vi "stations copy Station.vi"(7 "Connection Refnum":T1, 8 "error in (no error)":errorcluster, 9 "Stations Instruments":cluster{"Station Instruments":T2[]}[](array[cluster]), 10 "All Stations (empty)":T3[](array[typedef]), 11 "Station ID to Copy (\"\")":string) -> (0 "error out":errorcluster, 1 "Station Instruments":T2[](array[typedef]), 2 "Station Record":T3, 5 "Connection Refnum":T1)   [LabVIEW 2011]
uses:
  server/database/Stations/Station Record.ctl
  server/database/Stations/Instruments/Instrument Record.ctl
  Summitek EXT/ODBC/SQL Controls/Connection Refnum.ctl
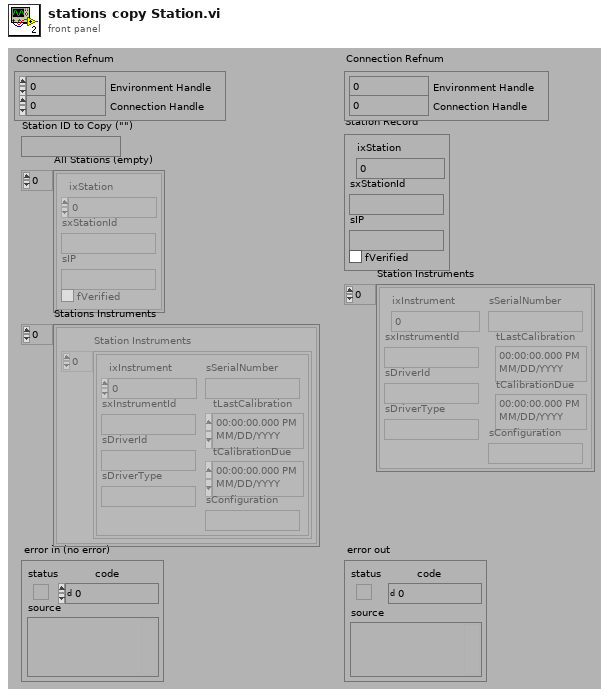
[diagram p1: front panel]
types:
  T1 = typedef "Connection Refnum.ctl" = cluster{"Environment Handle":i32, "Connection Handle":i32}
  T2 = typedef "Instrument Record.ctl" = cluster{"ixInstrument":i32, "sxInstrumentId":string, "sDriverId":string, "sDriverType":string, "sSerialNumber":string, "tLastCalibration":timestamp, "tCalibrationDue":timestamp, "sConfiguration":string}
  T3 = typedef "Station Record.ctl" = cluster{"ixStation":i32, "sxStationId":string, "sIP":string, "fVerified":bool}
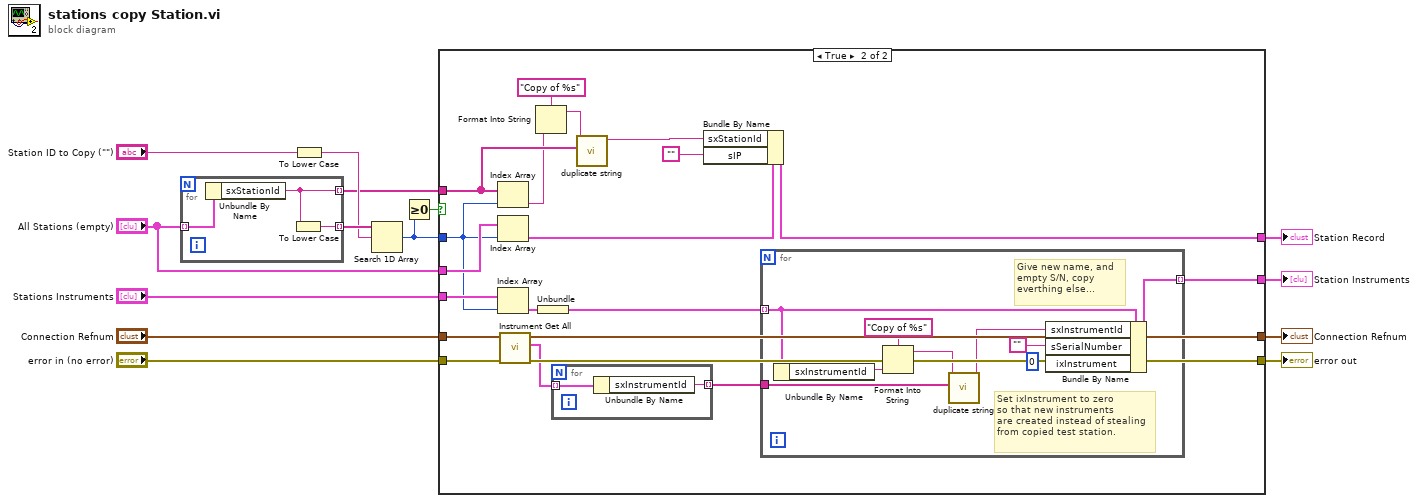
[diagram p0: block diagram]
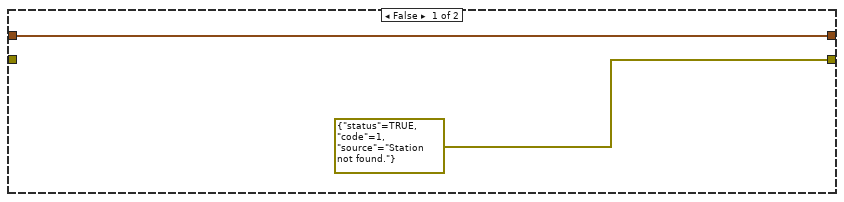
[diagram p2: hidden frame]
diagram:
  n1 = for {
    tunnel: "All Stations (empty)" -> [w17] mode=indexing
    tunnel: [w16] -> w14 mode=indexing
    tunnel: [w15] -> w4 mode=indexing
    n2 = Unbundle By Name(w17) -> ("sxStationId"=w15:string)
    n3 = To Lower Case(string=w15) -> (all lower case string=w16:string)
  }
  n4 = To Lower Case(string="Station ID to Copy (\"\")") -> (all lower case string=w13:string)
  n5 = Search 1D Array(1D array=w14, element=w13) -> (index of element=w11:i32)  [unwired: 1 out]
  n6 = Greater Or Equal To 0?(x=w11) -> (x >= 0?=w10:bool)
  n7 = case shown="True" w10 {
    tunnel: "All Stations (empty)" -> [_ w39]
    tunnel: w11 -> [_ w29]
    tunnel: [_ w37] -> w9
    tunnel: "error in (no error)" -> [_ w27]
    tunnel: [errorcluster {"status"=TRUE, "code"=1, "source"="Station not found."} ("error in (no error)") w26] -> w7
    tunnel: w4 -> [_ w34]
    tunnel: "Stations Instruments" -> [_ w30]
    tunnel: "Connection Refnum" -> [w18 w25]
    tunnel: [w18 w24] -> w2
    tunnel: [_ w20] -> w1
    frame False {
    }
    frame True {
      n8 = Index Array(array=w34, index=w29) -> (element=w33:string)
      n9 = Index Array(array=w39, index=w29) -> (element=w38:T3)
      n10 = Index Array(array=w30, index=w29) -> (element=w28:cluster{"Station Instruments":T2[]})
      n11 = call "Instrument Get All.vi"("error in (no error)"=w27, "Connection Refnum"=w25) -> ("error out"=w26:errorcluster, "Instruments"=w22:T2[], "Connection Refnum"=w24:T1)  [unwired: 2 in, 5 out]
      n12 = Format Into String(format string="Copy of %s", w33) -> (resulting string=w36:string)  [unwired: 2 in, 1 out]
      n13 = Unbundle(w28) -> ("Station Instruments"=w23:T2[])
      n14 = for {
        tunnel: w22 -> [w41] mode=indexing
        tunnel: [w40] -> w21 mode=indexing
        n15 = Unbundle By Name(w41) -> ("sxInstrumentId"=w40:string)
      }
      n16 = call "duplicate string.vi"("Array of Strings"=w34, "String"=w36) -> ("Updated String"=w32:string)  [unwired: 9 out]
      n17 = Bundle By Name(cluster=w38, "sxStationId"=w32, "sIP"="") -> (w37:T3)
      n18 = for {
        tunnel: w23 -> [w46] mode=indexing
        tunnel: w21 -> [w50]
        tunnel: [w43] -> w20 mode=indexing
        # "Set ixInstrument to zero\nso that new instruments\nare created instead of stealing\nfrom copied test station."
        # "Give new name, and\nempty S/N, copy\neverthing else..."
        n19 = Unbundle By Name(w46) -> ("sxInstrumentId"=w47:string)
        n20 = Format Into String(format string="Copy of %s", w47) -> (resulting string=w48:string)  [unwired: 2 in, 1 out]
        n21 = call "duplicate string.vi"("Array of Strings"=w50, "String"=w48) -> ("Updated String"=w45:string)  [unwired: 9 out]
        n22 = Bundle By Name(cluster=w46, "sxInstrumentId"=w45, "sSerialNumber"="", "ixInstrument"=0) -> (w43:T2)
      }
    }
  }
  "error out" <- w7
  "Station Record" <- w9
  "Station Instruments" <- w1
  "Connection Refnum" <- w2
